vi "Get_Data.vi"(0 "Add in":refnum<class "Add.lvclass">, 11 "Error In":errorcluster) -> (4 "Add out":refnum<class "Add.lvclass">, 15 "Error Out":errorcluster)   [LabVIEW 2020, in "Add.lvclass"]
doc: "Method to get the object data from the UI method."
uses:
  Add.lvclass
  D:/Github Projects/LV_Assignment/Tasks/A18/A18/Classes/Arithmetic_Operations/Arithmetic_Operations.lvclass
  Arithmetic_Operations/Arithmetic_Operations.lvclass
  Add.lvclass/Add.ctl
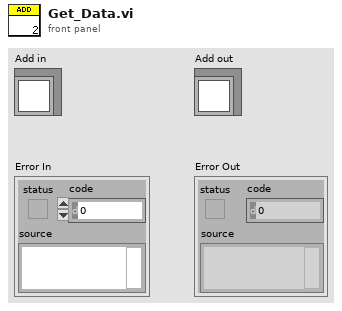
[diagram p1: front panel]
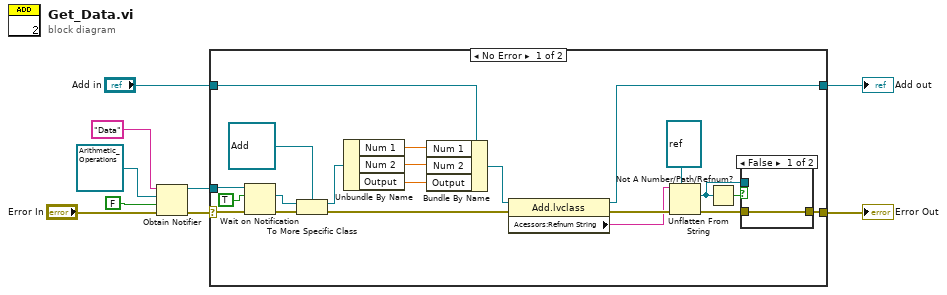
[diagram p0: block diagram]
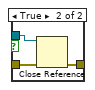
[diagram p2: hidden frame]
diagram:
  n1 = Obtain Notifier(name (unnamed)="Data", notification data type=refnum<class "Arithmetic_Operations.lvclass"> refnum ("Arithmetic_Operations.lvclass"), create if not found? (T)=FALSE, error in (no error)="Error In") -> (notifier out=w6:refnum<notifier>, error out=w4:errorcluster)  [unwired: 1 out]
  n2 = case shown="No Error" w4 {
    selector: w4 -> [w26 w36]
    tunnel: [w17 w36] -> w9
    tunnel: [w18 w35] -> w1
    tunnel: "Add in" -> [w30 w35]
    tunnel: w6 -> [w24 _]
    frame No Error {
      n3 = Wait on Notification(notifier=w24, ignore previous (F)=TRUE, error in (no error)=w26) -> (notification=w23:refnum<class "Arithmetic_Operations.lvclass">, error out=w25:errorcluster)  [unwired: 1 in, 2 out]
      n4 = To More Specific Class(target class=refnum<class "Add.lvclass"> refnum ("Add.lvclass"), reference=w23, error in=w25) -> (specific class reference=w22:refnum<class "Add.lvclass">, error out=w16:errorcluster)
      n5 = Unbundle By Name(w22) -> ("Num 1"=w29:dbl, "Num 2"=w28:dbl, "Output"=w27:dbl)
      n6 = Bundle By Name(cluster=w30, "Num 1"=w29, "Num 2"=w28, "Output"=w27) -> (w19:refnum<class "Add.lvclass">)
      n7 = property class="Add.lvclass"(reference=w19, error in=w16) -> (reference out=w18:refnum<class "Add.lvclass">, error out=w15:errorcluster, "Acessors:Refnum String"=w14:string)
      n8 = Unflatten From String(type=refnum<vi> refnum ("reference out"), binary string=w14, error in (no error)=w15) -> (value=w10:refnum<vi>, error out=w13:errorcluster)  [unwired: 2 in, 1 out]
      n9 = Not A Number/Path/Refnum?(number/path/refnum=w10) -> (NaN/Path/Refnum?=w11:bool)
      n10 = case shown="False" w11 {
        tunnel: [w31 w34] -> w17
        tunnel: w13 -> [w31 w33]
        tunnel: w10 -> [_ w32]
        frame False {
        }
        frame True {
          n11 = Close Reference(reference=w32, error in (no error)=w33) -> (error out=w34:errorcluster)
        }
      }
    }
    frame Error {
    }
  }
  "Error Out" <- w9
  "Add out" <- w1
